vi "Simple Triangle Waveform.vi"(6 "delta t":dbl=1.0, 7 "amplitude":dbl=1.0, 9 "n cycles":dbl=1.0, 10 "t0":dbl=-1.0, 11 "offset":dbl) -> (3 "triangle waveform":waveform(dbl))   [LabVIEW 2023]
doc: "Produces a triangle wave."
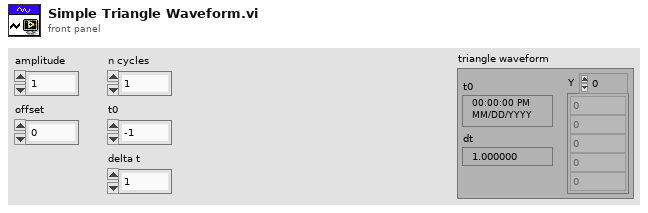
[diagram p1: front panel]
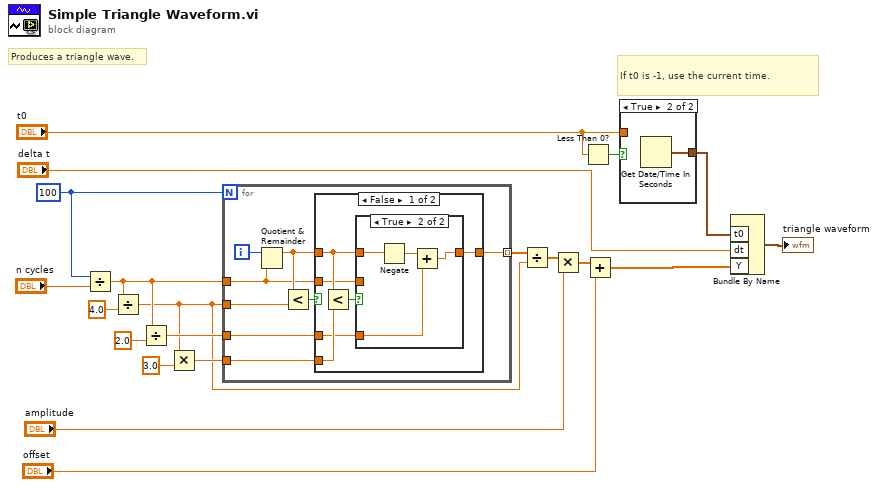
[diagram p0: block diagram]
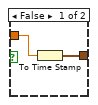
[diagram p2: hidden frame]
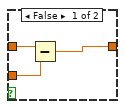
[diagram p3: hidden frame]
diagram:
  w15 = 100 ("n points")
  # "If t0 is -1, use the current time."
  # "Produces a triangle wave."
  n1 = Divide(x=w15, y="n cycles") -> (x/y=w10:dbl)
  n2 = Divide(x=w10, y=4.0) -> (x/y=w8:dbl)
  n3 = Divide(x=w10, y=2.0) -> (x/y=w9:dbl)
  n4 = Multiply(x=w8, y=3.0) -> (x*y=w13:dbl)
  n5 = for {
    N: w15 -> [_]
    tunnel: w10 -> [w23]
    tunnel: w8 -> [w22]
    tunnel: [w25] -> w11 mode=indexing
    tunnel: w13 -> [w24]
    tunnel: w9 -> [w21]
    i -> [w28]
    n6 = Quotient & Remainder(x=w28, y=w23) -> (x-y*floor(x/y)=w26:dbl)  [unwired: 1 out]
    n7 = Less?(x=w26, y=w22) -> (x < y?=w27:bool)
    n8 = case shown="False" w27 {
      tunnel: [w31 w42] -> w25
      tunnel: w26 -> [w32 w42]
      tunnel: w24 -> [w33 _]
      tunnel: w23 -> [w30 _]
      tunnel: w21 -> [w29 _]
      frame False {
        n9 = Less?(x=w32, y=w33) -> (x < y?=w34:bool)
        n10 = case shown="True" w34 {
          tunnel: w32 -> [w37 w41]
          tunnel: [w35 w39] -> w31
          tunnel: w30 -> [w36 _]
          tunnel: w29 -> [_ w38]
          frame False {
            n11 = Subtract(x=w37, y=w36) -> (x-y=w35:dbl)
          }
          frame True {
            n12 = Negate(x=w41) -> (-x=w40:dbl)
            n13 = Add(x=w40, y=w38) -> (x+y=w39:dbl)
          }
        }
      }
      frame True {
      }
    }
  }
  n14 = Divide(x=w11, y=w8) -> (x/y=w12:dbl[])
  n15 = Multiply(x=w12, y="amplitude") -> (x*y=w18:dbl[])
  n16 = Less Than 0?(x="t0") -> (x < 0?=w4:bool)
  n17 = Add(x=w18, y="offset") -> (x+y=w16:dbl[])
  n18 = case shown="True" w4 {
    tunnel: [w44 w45] -> w2
    tunnel: "t0" -> [w43 _]
    frame False {
      n19 = To Time Stamp(1:w43) -> (0:w44:timestamp)
    }
    frame True {
      n20 = Get Date/Time In Seconds() -> (seconds since 1Jan1904=w45:timestamp)
    }
  }
  n21 = Bundle By Name("t0"=w2, "dt"="delta t", "Y"=w16) -> (→"triangle waveform":waveform(dbl))  [unwired: 1 in]
